vi "Cargo Manip Control.vi"   [LabVIEW 2018]
uses:
  SubSystems/Cargo Intake/Cargo Intake Global.vi
  SubSystems/Controllers/Manipulator Controlller/Manipulator Controller Global.vi
  SubSystems/Robot Information/Robot Information Global.vi
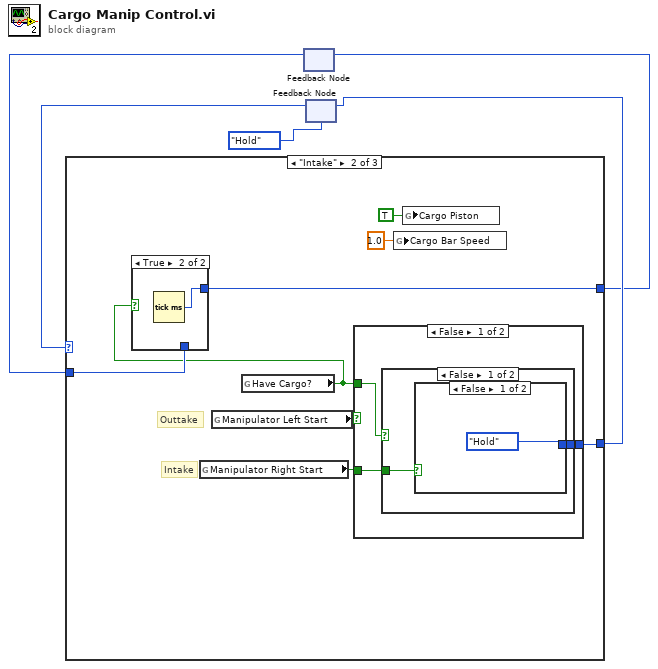
[diagram p0: block diagram]
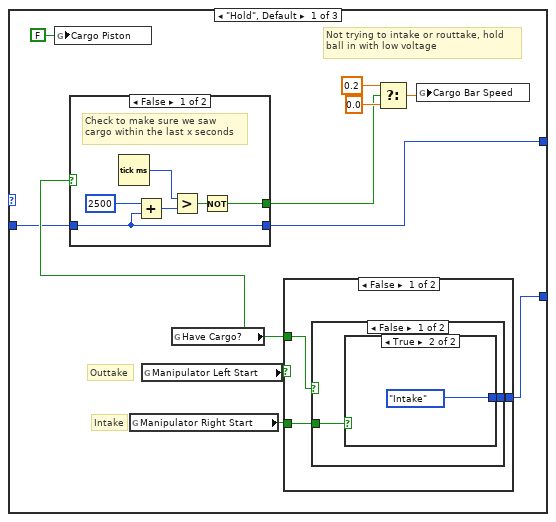
[diagram p2: hidden frame]
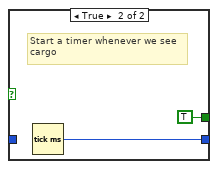
[diagram p3: hidden frame]
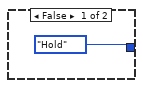
[diagram p4: hidden frame]
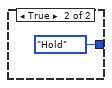
[diagram p5: hidden frame]
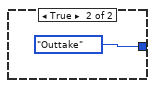
[diagram p6: hidden frame]
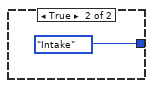
[diagram p8: hidden frame]
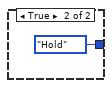
[diagram p9: hidden frame]
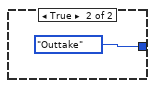
[diagram p10: hidden frame]
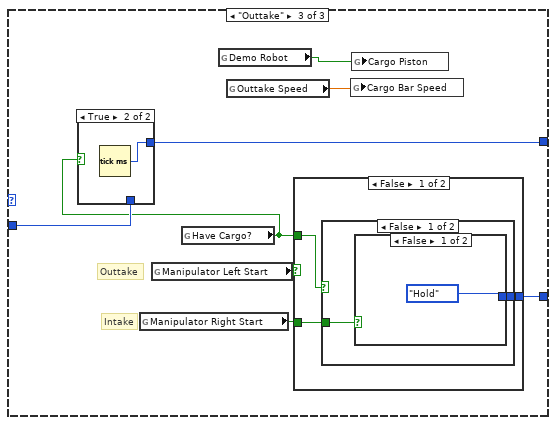
[diagram p11: hidden frame]
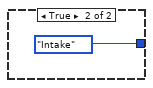
[diagram p13: hidden frame]
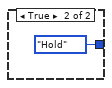
[diagram p14: hidden frame]
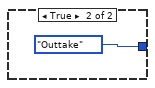
[diagram p15: hidden frame]
diagram:
  n1 = feedback #1() -> (w1:u32)  [unwired: 1 in]
  n2 = feedback #2(enum16{"Going Up", "Outtake", "Intake", "Hold"}."Hold") -> (w4:enum16{"Going Up", "Outtake", "Intake", "Hold"})
  n3 = case shown="\"Intake\"" w4 {
    tunnel: [w14 w37 w58] -> w3
    tunnel: [w9 w35 w56] -> w2
    tunnel: w1 -> [w7 w36 w57]
    frame "Hold", Default {
      # "Outtake"
      # "Intake"
      # "Not trying to intake or routtake, hold\nball in with low voltage"
      n4 = global write "Cargo Intake Global.vi" "Cargo Piston"(FALSE ("Cargo Piston")) -> ()
      n5 = global read "Manipulator Controller Global.vi" "Manipulator Right Start"() -> (w16:bool)
      n6 = global read "Manipulator Controller Global.vi" "Manipulator Left Start"() -> (w15:bool)
      n7 = global read "Cargo Intake Global.vi" "Have Cargo?"() -> (w8:bool)
      n8 = case shown="False" w8 {
        tunnel: [w22 w24] -> w9
        tunnel: w7 -> [w22 _]
        tunnel: [w17 TRUE] -> w6
        frame False {
          # "Check to make sure we saw \ncargo within the last x seconds"
          n9 = Tick Count (ms)() -> (millisecond timer value=w19:u32)
          n10 = Add(x=u32 2500, y=w22) -> (x+y=w20:u32)
          n11 = Greater?(x=w19, y=w20) -> (0:w18:bool)
          n12 = Not(x=w18) -> (.not. x?=w17:bool)
        }
        frame True {
          # "Start a timer whenever we see\ncargo"
          n13 = Tick Count (ms)() -> (millisecond timer value=w24:u32)
        }
      }
      n14 = case shown="False" w15 {
        tunnel: w16 -> [w27 _]
        tunnel: [w26 enum16{"Going Up", "Outtake", "Intake", "Hold"}."Outtake"] -> w14
        tunnel: w8 -> [w25 _]
        frame False {
          n15 = case shown="False" w25 {
            tunnel: w27 -> [w29 _]
            tunnel: [w28 enum16{"Going Up", "Outtake", "Intake", "Hold"}."Hold"] -> w26
            frame False {
              n16 = case shown="True" w29 {
                tunnel: [enum16{"Going Up", "Outtake", "Intake", "Hold"}."Hold" enum16{"Going Up", "Outtake", "Intake", "Hold"}."Intake"] -> w28
                frame False {
                }
                frame True {
                }
              }
            }
            frame True {
            }
          }
        }
        frame True {
        }
      }
      n17 = Select(t=0.2, s=w6, f=0.0) -> (s? t:f=w12:dbl)
      n18 = global write "Cargo Intake Global.vi" "Cargo Bar Speed"(w12) -> ()
    }
    frame "Intake" {
      # "Outtake"
      # "Intake"
      n19 = global read "Manipulator Controller Global.vi" "Manipulator Right Start"() -> (w41:bool)
      n20 = global read "Manipulator Controller Global.vi" "Manipulator Left Start"() -> (w40:bool)
      n21 = global read "Cargo Intake Global.vi" "Have Cargo?"() -> (w34:bool)
      n22 = case shown="True" w34 {
        tunnel: w36 -> [w42 _]
        tunnel: [w42 w43] -> w35
        frame False {
        }
        frame True {
          n23 = Tick Count (ms)() -> (millisecond timer value=w43:u32)
        }
      }
      n24 = case shown="False" w40 {
        tunnel: w41 -> [w46 _]
        tunnel: [w45 enum16{"Going Up", "Outtake", "Intake", "Hold"}."Outtake"] -> w37
        tunnel: w34 -> [w44 _]
        frame False {
          n25 = case shown="False" w44 {
            tunnel: w46 -> [w48 _]
            tunnel: [w47 enum16{"Going Up", "Outtake", "Intake", "Hold"}."Hold"] -> w45
            frame False {
              n26 = case shown="False" w48 {
                tunnel: [enum16{"Going Up", "Outtake", "Intake", "Hold"}."Hold" enum16{"Going Up", "Outtake", "Intake", "Hold"}."Intake"] -> w47
                frame False {
                }
                frame True {
                }
              }
            }
            frame True {
            }
          }
        }
        frame True {
        }
      }
      n27 = global write "Cargo Intake Global.vi" "Cargo Bar Speed"(1.0 ("Cargo Bar Speed")) -> ()
      n28 = global write "Cargo Intake Global.vi" "Cargo Piston"(TRUE ("Cargo Piston")) -> ()
    }
    frame "Outtake" {
      # "Outtake"
      # "Intake"
      n29 = global read "Manipulator Controller Global.vi" "Manipulator Right Start"() -> (w60:bool)
      n30 = global read "Manipulator Controller Global.vi" "Manipulator Left Start"() -> (w59:bool)
      n31 = global read "Cargo Intake Global.vi" "Have Cargo?"() -> (w55:bool)
      n32 = case shown="True" w55 {
        tunnel: w57 -> [w61 _]
        tunnel: [w61 w62] -> w56
        frame False {
        }
        frame True {
          n33 = Tick Count (ms)() -> (millisecond timer value=w62:u32)
        }
      }
      n34 = global read "Robot Information Global.vi" "Demo Robot"() -> (w53:bool)
      n35 = global read "Cargo Intake Global.vi" "Outtake Speed"() -> (w54:dbl)
      n36 = case shown="False" w59 {
        tunnel: w60 -> [w65 _]
        tunnel: [w64 enum16{"Going Up", "Outtake", "Intake", "Hold"}."Outtake"] -> w58
        tunnel: w55 -> [w63 _]
        frame False {
          n37 = case shown="False" w63 {
            tunnel: w65 -> [w67 _]
            tunnel: [w66 enum16{"Going Up", "Outtake", "Intake", "Hold"}."Hold"] -> w64
            frame False {
              n38 = case shown="False" w67 {
                tunnel: [enum16{"Going Up", "Outtake", "Intake", "Hold"}."Hold" enum16{"Going Up", "Outtake", "Intake", "Hold"}."Intake"] -> w66
                frame False {
                }
                frame True {
                }
              }
            }
            frame True {
            }
          }
        }
        frame True {
        }
      }
      n39 = global write "Cargo Intake Global.vi" "Cargo Bar Speed"(w54) -> ()
      n40 = global write "Cargo Intake Global.vi" "Cargo Piston"(w53) -> ()
    }
  }
  n41 = feedback-in #1(w2) -> ()
  n42 = feedback-in #2(w3) -> ()
